vi "Go to COOKING.vi"(8 "error in (no error)":errorcluster, 11 "COOKING in":refnum<class "COOKING.lvclass">) -> (0 "error out":errorcluster, 3 "State Actor.lvclass":refnum<class "State Actor.lvclass">)   [LabVIEW 2024, in "Chef States.lvlib" / "COOKING.lvclass"]
uses:
  COOKING.lvclass
  <vilib>/NI/Actors/State Actor/State Actor/State Actor.lvclass
  COOKING.lvclass/COOKING.ctl
  C:/Users/burakkorkmaz/Desktop/Leveling/repo/Chef States/Chef State/Chef State.lvclass
  C:/Program Files/National Instruments/LabVIEW 2024/vi.lib/NI/Actors/State Actor/State Actor/State Actor.lvclass
  C:/Program Files/National Instruments/LabVIEW 2024/vi.lib/ActorFramework/Actor/Actor.lvclass
  C:/Users/burakkorkmaz/Desktop/Leveling/repo/Chef States/COOKING/COOKING.lvclass
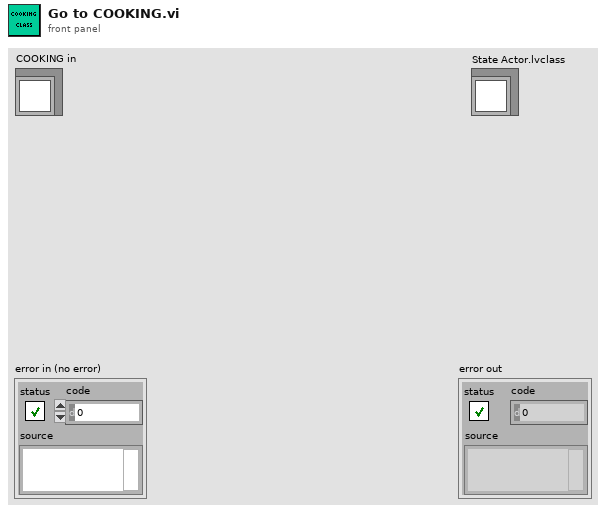
[diagram p1: front panel]
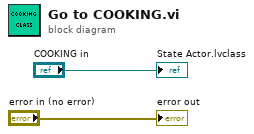
[diagram p0: block diagram]
diagram:
  "error out" <- "error in (no error)"
  "State Actor.lvclass" <- "COOKING in"
